vi "Linear Ramp by Number (CDB).vi"(6 "Options":T1=enum."Include Both Ends", 9 "# Steps":i32=1, 10 "End":cdb=1.0+0.0i, 11 "Start":cdb) -> (1 "# Elements":i32, 3 "Ramp":cdb[](array[numeric]))   [LabVIEW 2019]
doc: "Creates a linear ramp with steps provided by \"Delta\".\nDepending on the chosen Options:\n\n- Include Min/Exclude Max (Default)\n- Exclude Min/Include Max\n- Include Both\n- Exclude Both\n\nthe number of array elements will vary as well as the start and end values."
uses:
  Linear Ramp End Options.ctl
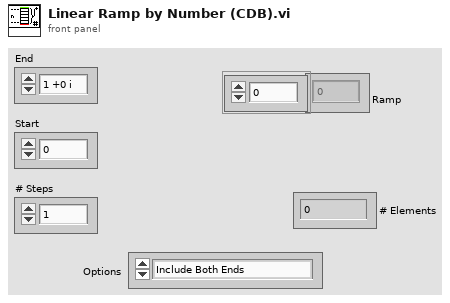
[diagram p1: front panel]
types:
  T1 = typedef "Linear Ramp End Options.ctl" = enum16{"Include Min/Exclude Max", "Exclude Min/Include Max", "Include Both Ends", "Exclude Both Ends"}
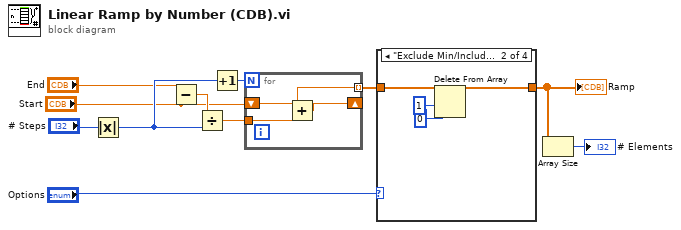
[diagram p0: block diagram]
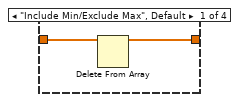
[diagram p2: hidden frame]
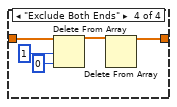
[diagram p4: hidden frame]
diagram:
  n1 = Absolute Value(x="# Steps") -> (abs(x)=w8:i32)
  n2 = Subtract(x="End", y="Start") -> (x-y=w10:cdb)
  n3 = Divide(x=w10, y=w8) -> (x/y=w9:cdb)
  n4 = Increment(x=w8) -> (x+1=w7:i32)
  n5 = for {
    N: w7 -> [_]
    shift-right: [w13] -> _
    shift-left: "Start" -> [w12]
    tunnel: w9 -> [w14]
    tunnel: [w12] -> w5 mode=indexing
    n6 = Add(x=w12, y=w14) -> (x+y=w13:cdb)
  }
  n7 = case shown="\"Exclude Min/Include Max\"" "Options" {
    tunnel: w5 -> [w16 w20 w21 w26]
    tunnel: [w15 w19 w21 w22] -> w3
    frame "Include Min/Exclude Max", Default {
      n8 = Delete From Array(array=w16) -> (array with subset deleted=w15:cdb[])  [unwired: 2 in, 1 out]
    }
    frame "Exclude Min/Include Max" {
      n9 = Delete From Array(array=w20, length=1, index=0) -> (array with subset deleted=w19:cdb[])  [unwired: 1 out]
    }
    frame "Include Both Ends" {
    }
    frame "Exclude Both Ends" {
      n10 = Delete From Array(array=w26, length=1, index=0) -> (array with subset deleted=w25:cdb[])  [unwired: 1 out]
      n11 = Delete From Array(array=w25) -> (array with subset deleted=w22:cdb[])  [unwired: 2 in, 1 out]
    }
  }
  "Ramp" <- w3
  n12 = Array Size(array=w3) -> (size(s)=→"# Elements":i32)
